vi "Initialize.vi"(8 "error in":errorcluster, 10 "InstanceName":string, 11 "ChillerNew.lvclass":refnum<class "ChillerNew.lvclass">) -> (0 "error out":errorcluster, 3 "output cluster":refnum<class "ChillerNew.lvclass">)   [LabVIEW 2023, in "ChillerNew.lvclass"]
uses:
  ChillerNew.lvclass
  ChillerNew.lvclass/ChillerNew.ctl
  Utilities/Utilities.lvlib
  <vilib>/ADAS Replay HIL/Channels/Tag Wrapper/Tag Wrapper.lvlib
  <vilib>/ADAS Replay HIL/Channels/Tag Wrapper/Polymorphic/Open Consumer Tag (Cluster).vi
  <vilib>/ADAS Replay HIL/Channels/Tag Wrapper/Polymorphic/Open Producer Tag (Cluster).vi
  b9c13089-0281-44b9-a90f-aec73f88b65c.vi
  248f2659-eb42-462d-9a15-8e5b3aec119f.vi
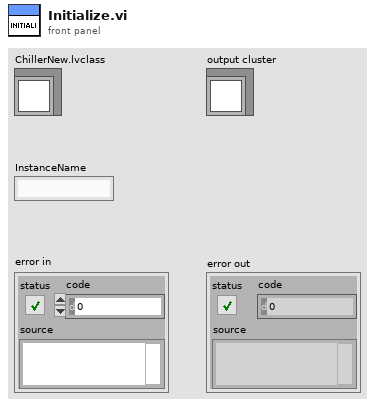
[diagram p1: front panel]
types:
  T1 = cluster{"OnOffCtl":bool, "SP1":dbl, "Watchdog":i32}
  T2 = cluster{"OnOffSts":bool, "AV1":dbl, "WatchdogSTS":i32}
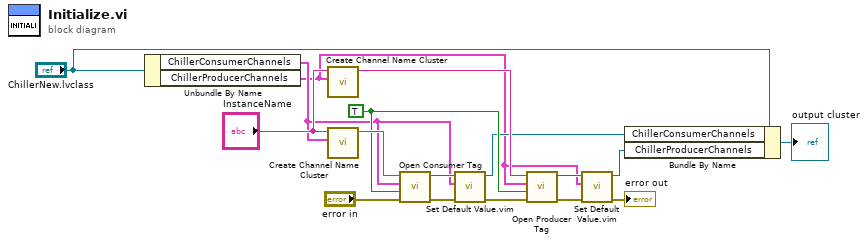
[diagram p0: block diagram]
diagram:
  w12 = TRUE ("Create if not found? (T)")
  n1 = Unbundle By Name("ChillerNew.lvclass") -> ("ChillerConsumerChannels"=w8:T1, "ChillerProducerChannels"=w1:T2)
  n2 = call "Create Channel Name Cluster.vi"("Cluster"=w1, "Instance Name"="InstanceName") -> ("Data Channel Name"=w11:string)  [unwired: 8 in, 1 out]
  n3 = call "Create Channel Name Cluster.vi"("Cluster"=w8, "Instance Name"="InstanceName") -> ("Data Channel Name"=w14:string)  [unwired: 8 in, 1 out]
  n4 = call-poly <vilib>:"Open Consumer Tag.vi"("error in"="error in", "Create if not found? (T)"=w12, "Cluster"=w8, "Channel Name"=w14) -> ("error out"=w7:errorcluster, "ADAS HIL Channel"=w10:refnum<k21>)  [unwired: 6 in]
  n5 = call "Set Default Value.vim"("error in"=w7, "Data in"=w8, "ADAS HIL Channel in"=w10) -> ("error out"=w6:errorcluster, "ADAS HIL Channel out"=w9:refnum<k21>)  [unwired: 7 in]
  n6 = call-poly <vilib>:"Open Producer Tag.vi"("error in"=w6, "Create if not found? (T)"=w12, "Cluster"=w1, "Channel Name"=w11) -> ("error out"=w5:errorcluster, "ADAS HIL Channel"=w3:refnum<k21>)  [unwired: 6 in]
  n7 = call "Set Default Value.vim"("error in"=w5, "Data in"=w1, "ADAS HIL Channel in"=w3) -> ("error out"=→"error out":errorcluster, "ADAS HIL Channel out"=w2:refnum<k21>)  [unwired: 7 in]
  n8 = Bundle By Name(cluster="ChillerNew.lvclass", "ChillerConsumerChannels"=w9, "ChillerProducerChannels"=w2) -> (→"output cluster":refnum<class "ChillerNew.lvclass">)
